vi "ble_search_handle_by_service_and_characteristic.vi"(8 "error in (no error)":errorcluster, 9 "Characteristic UUID":string, 10 "Service UUID":string, 11 "Handle table":string[][](array[string])) -> (0 "error out":errorcluster, 2 "Handle":string)   [LabVIEW 2015]
panel:
  out "unsigned byte array":u8[](array[numeric])
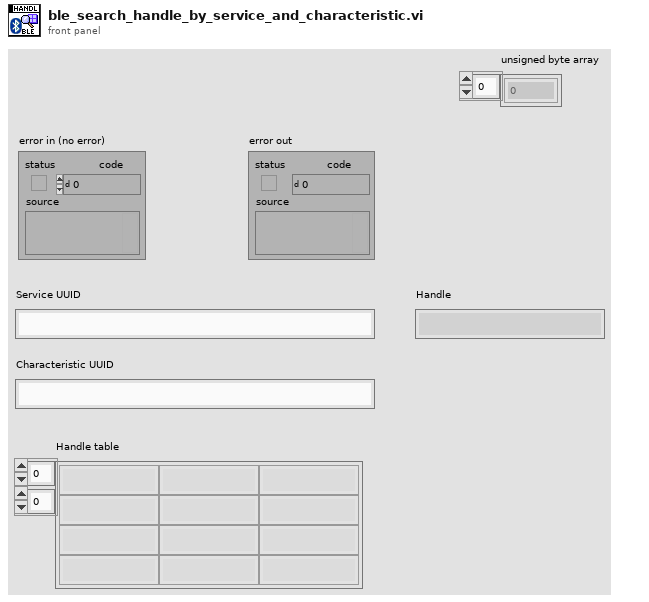
[diagram p1: front panel]
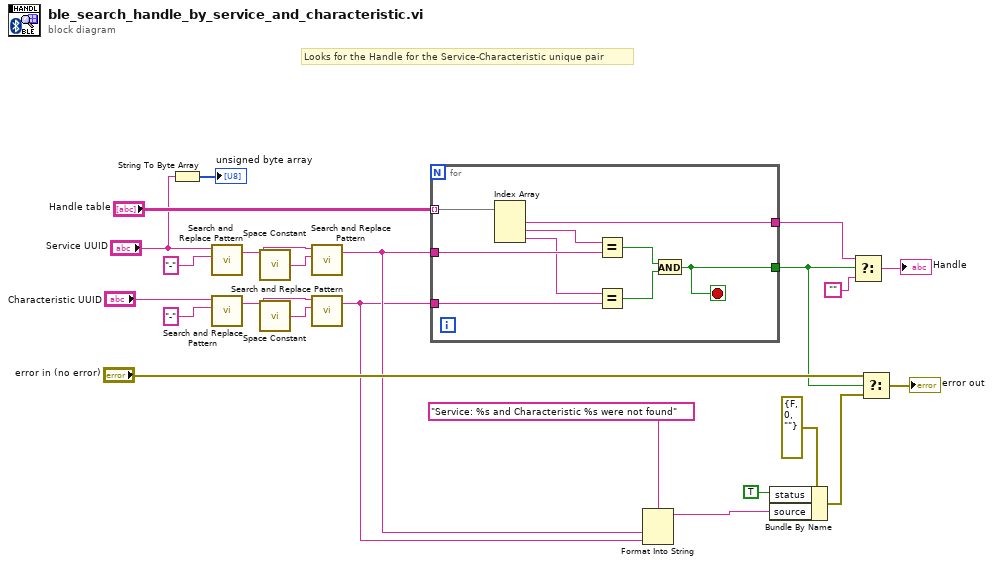
[diagram p0: block diagram]
diagram:
  # "Looks for the Handle for the Service-Characteristic unique pair"
  n1 = String To Byte Array(string="Service UUID") -> (unsigned byte array=→"unsigned byte array":u8[])
  n2 = call <vilib>:"Search and Replace Pattern.vi"("string"="Service UUID", "regular expression (\"\")"="-" ("regular expression (\"\")")) -> ("result string"=w21:string)  [unwired: 3 in, 1 out]
  n3 = call <vilib>:"Search and Replace Pattern.vi"("string"="Characteristic UUID", "regular expression (\"\")"="-" ("regular expression (\"\")")) -> ("result string"=w20:string)  [unwired: 3 in, 1 out]
  n4 = call <vilib>:"Space Constant.vi"() -> ("String"=w22:string)
  n5 = call <vilib>:"Space Constant.vi"() -> ("String"=w19:string)
  n6 = call <vilib>:"Search and Replace Pattern.vi"("string"=w21, "regular expression (\"\")"=w22) -> ("result string"=w9:string)  [unwired: 3 in, 1 out]
  n7 = call <vilib>:"Search and Replace Pattern.vi"("string"=w20, "regular expression (\"\")"=w19) -> ("result string"=w8:string)  [unwired: 3 in, 1 out]
  n8 = for {
    tunnel: "Handle table" -> [w32] mode=indexing
    tunnel: [w31] -> w6
    tunnel: w9 -> [w29]
    tunnel: w8 -> [w28]
    tunnel: [w24] -> w3
    stop <- w24 stop-if-true
    n9 = Index Array(array=w32) -> (element #1=w31:string, element #2=w30:string, element #3=w27:string)  [unwired: 3 in]
    n10 = Equal?(x=w30, y=w29) -> (x = y?=w26:bool)
    n11 = Equal?(x=w27, y=w28) -> (x = y?=w25:bool)
    n12 = And(x=w26, y=w25) -> (x .and. y?=w24:bool)
  }
  n13 = Format Into String(format string="Service: %s and Characteristic %s were not found", w9, w8) -> (resulting string=w10:string)  [unwired: 2 in, 1 out]
  n14 = Bundle By Name(cluster=errorcluster {"status"=FALSE, "code"=0, "source"=""} ("error in (no error)"), "status"=TRUE, "source"=w10) -> (w13:errorcluster)
  n15 = Select(t=w6, s=w3, f="") -> (s? t:f=→"Handle":string)
  n16 = Select(t="error in (no error)", s=w3, f=w13) -> (s? t:f=→"error out":errorcluster)
